vi "Start log.vi"(8 "error in (no error)":errorcluster, 10 "Filename root":string="instrinsic", 11 "Relative path":string="DATA_LOGS") -> (0 "error out":errorcluster, 1 "Logging":bool, 3 "Byte Stream File out":refnum<file>)   [LabVIEW 2016]
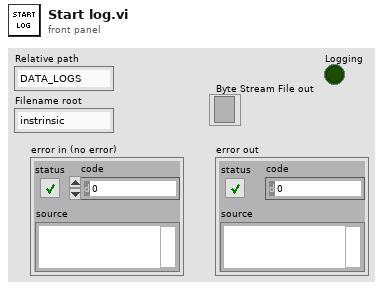
[diagram p1: front panel]
types:
  T1 = enum16{"open", "replace", "create", "open or create", "replace or create", "replace or create with confirmation"}
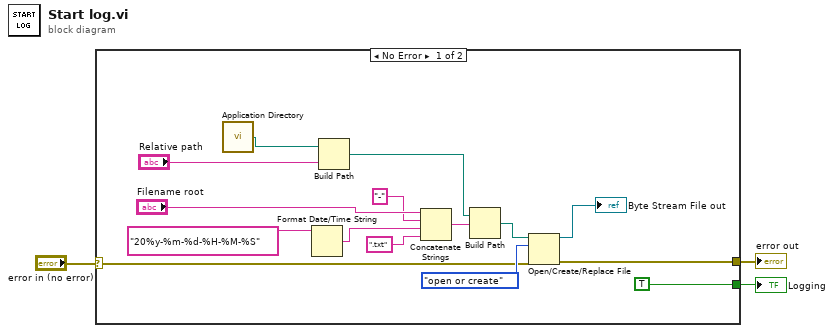
[diagram p0: block diagram]
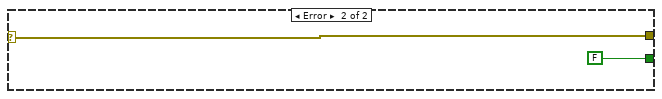
[diagram p2: hidden frame]
diagram:
  n1 = case shown="No Error" "error in (no error)" {
    selector: "error in (no error)" -> [w9 w20]
    tunnel: [w8 w20] -> w3
    tunnel: [TRUE FALSE] -> w1
    frame No Error {
      n2 = call <vilib>:"Application Directory.vi"() -> ("Application Directory"=w4:path)
      n3 = Format Date/Time String(time format string (%c)="20%y-%m-%d-%H-%M-%S") -> (date/time string=w11:string)  [unwired: 2 in]
      n4 = Build Path(base path=w4, name or relative path="Relative path") -> (appended path=w5:path)
      n5 = Concatenate Strings("Filename root", "-", w11, ".txt") -> (w14:string)
      n6 = Build Path(base path=w5, name or relative path=w14) -> (appended path=w15:path)
      n7 = Open/Create/Replace File(file path (use dialog)=w15, error in=w9, operation (0:open)=T1."open or create") -> (refnum out=→"Byte Stream File out":refnum<file>, error out=w8:errorcluster)  [unwired: 3 in, 1 out]
    }
    frame Error {
    }
  }
  "error out" <- w3
  "Logging" <- w1
